vi "basic_Coerce Phase Angle.vi"(4 "Phase Angle":dbl) -> (1 "Phase Angle (-180 to 180)":dbl)   [LabVIEW 2011, in "NI_EP_Basic.lvlib"]
uses:
  <vilib>/addons/Electrical Power/Basic/NI_EP_Basic.lvlib
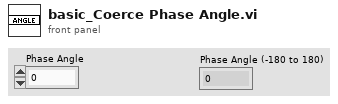
[diagram p1: front panel]
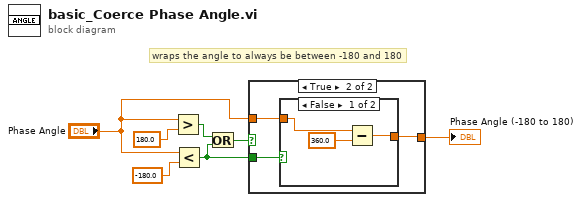
[diagram p0: block diagram]
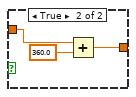
[diagram p3: hidden frame]
diagram:
  # "wraps the angle to always be between -180 and 180"
  n1 = Greater?(x="Phase Angle", y=180.0 ("x")) -> (0:w7:bool)
  n2 = Less?(x="Phase Angle", y=-180.0 ("x")) -> (x < y?=w4:bool)
  n3 = Or(x=w7, y=w4) -> (x .or. y?=w6:bool)
  n4 = case shown="True" w6 {
    tunnel: "Phase Angle" -> [w8 w10]
    tunnel: [w8 w9] -> w5
    tunnel: w4 -> [_ w11]
    frame False {
    }
    frame True {
      n5 = case shown="False" w11 {
        tunnel: w10 -> [w13 w17]
        tunnel: [w14 w16] -> w9
        frame False {
          n6 = Subtract(x=w13, y=360.0) -> (x-y=w14:dbl)
        }
        frame True {
          n7 = Add(x=w17, y=360.0) -> (x+y=w16:dbl)
        }
      }
    }
  }
  "Phase Angle (-180 to 180)" <- w5
